vi "AMB_Dual_Interface_Setup.vi"(0 "ABM":i16, 1 "TCP":bool, 2 "CAN Port In":string="CAN0", 3 "Port#":u16, 4 "Host":string) -> (5 "CAN Network\nObject \nHandle Out":u32, 6 "error out":errorcluster {"code" format="%.0x"})   [LabVIEW 2017]
doc: "Opens and sets up a NI-CAN interface board for use as an AMB master.\nThe CAN Port terminal defaults to CAN0."
uses:
  <vilib>/nican/nican.llb/ncNetAttr.ctl
  AMB_Global.gbl.vi
panel:
  in  "CAN Network Interface Config Cluster":T1={"Start On Open"=enum."TRUE", "Baud Rate"=1000000, "Read Queue Length"=10, "Write Queue Length"=10, "Standard Comparator"=0, "Standard Mask"=0, "Extended Comparator"=0, "Extended Mask"=0} {"Baud Rate" min=5000 max=1333333 step=1; "Extended Mask" format="%.0x"; "Extended Comparator" format="%.0x"; "Standard Mask" format="%.0x"; "Standard Comparator" format="%.0x"; "Write Queue Length" max=1000; "Read Queue Length" max=1000}
  # "ALMA Monitor and Control Bus\nSetup Bus"
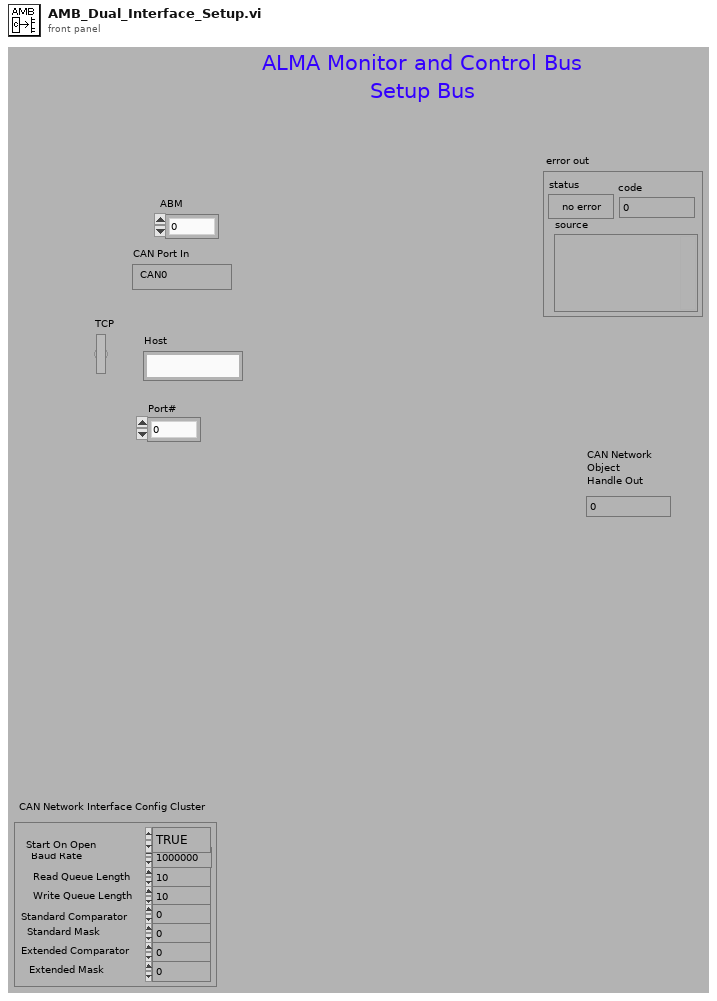
[diagram p1: front panel]
types:
  T1 = typedef "ncNetAttr.ctl" = cluster{"Start On Open":enum32{"FALSE", "TRUE"}, "Baud Rate":u32, "Read Queue Length":u32, "Write Queue Length":u32, "Standard Comparator":u32, "Standard Mask":u32, "Extended Comparator":u32, "Extended Mask":u32}
  T2 = typedef "xobjhandle.ctl" = u32
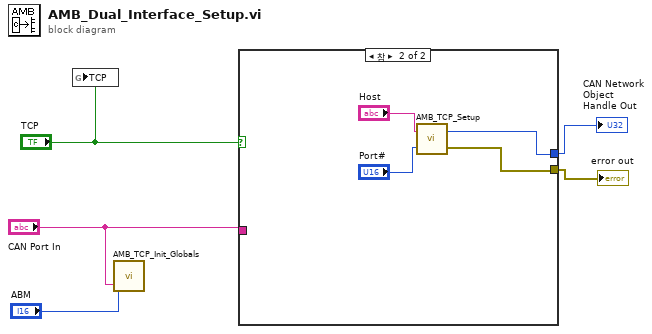
[diagram p0: block diagram]
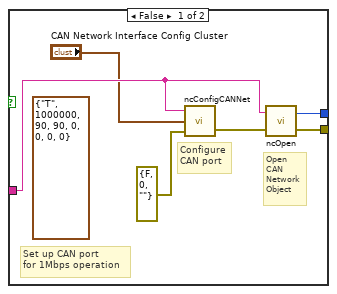
[diagram p2: hidden frame]
diagram:
  n1 = global write "AMB_Global.gbl.vi" "TCP"("TCP") -> ()
  n2 = call "AMB_TCP_Init_Globals.vi"("CAN Port In"="CAN Port In", "ABM In"="ABM") -> ()  [unwired: 1 in, 1 out]
  n3 = case shown="참" "TCP" {
    tunnel: "CAN Port In" -> [w10 _]
    tunnel: [w9 w12] -> w4
    tunnel: [w8 w13] -> w3
    frame False {
      (unwired) T1 {"Start On Open"=enum."TRUE", "Baud Rate"=1000000, "Read Queue Length"=90, "Write Queue Length"=90, "Standard Comparator"=0, "Standard Mask"=0, "Extended Comparator"=0, "Extended Mask"=0} ("ConfigCluster")
      # "Set up CAN port\nfor 1Mbps operation"
      # "Configure\nCAN port"
      # "Open\nCAN\nNetwork\nObject"
      n4 = call <vilib>:"ncConfigCANNet.vi"("Error in"=errorcluster {"status"=FALSE, "code"=0, "source"=""}, "CAN Network Interface Config"="CAN Network Interface Config Cluster", "ObjName"=w10) -> ("Error out"=w11:errorcluster)  [unwired: 2 in]
      n5 = call <vilib>:"ncOpen.vi"("Error in"=w11, "ObjName"=w10) -> ("Error out"=w8:errorcluster, "ObjHandle out"=w9:T2)
    }
    frame True {
      n6 = call "AMB_TCP_Setup.vi"("Host IP"="Host", "Port #"="Port#") -> ("TCP Refnum"=w12:u32, "error out"=w13:errorcluster)  [unwired: 1 in]
    }
  }
  "CAN Network\nObject \nHandle Out" <- w4
  "error out" <- w3
